vi "Get Package Details.vi"(7 "LabVIEW Web Service Request":refnum<class "Web Request.lvclass">) -> ()   [LabVIEW 2020]
uses:
  <vilib>/wsapi/Web Request.lvclass
  Libraries/Packages/Repo_class/Repo.lvclass/Repo.ctl
  Libraries/Packages/Package_class/Package.lvclass/Package.ctl
  Libraries/Packages/Package Version_class/Package Version.lvclass/Package Version.ctl
  Libraries/Packages/Package Version_class/Read Version.vi
  Libraries/Packages/Package_class/Read Versions.vi
  Libraries/Packages/Package_class/Read Name.vi
  Libraries/Packages/Repo_class/Read Packages.vi
  Libraries/WSsupport/GV_Repos.vi
  Libraries/Packages/Package_class/Package.lvclass
  Libraries/Packages/Package Version_class/Package Version.lvclass
  Libraries/WSsupport/WSsupport.lvlib
  Libraries/ServerErrors/ServerErrors.lvlib
  Libraries/Packages/Repo_class/Repo.lvclass
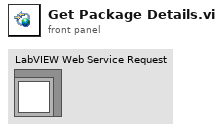
[diagram p1: front panel]
types:
  T1 = typedef "ServerErrors.lvlib/Error Message--cluster.ctl" = cluster{"HTTP Code":i32, "JSON Response":cluster{"error":string, "reason":string}}
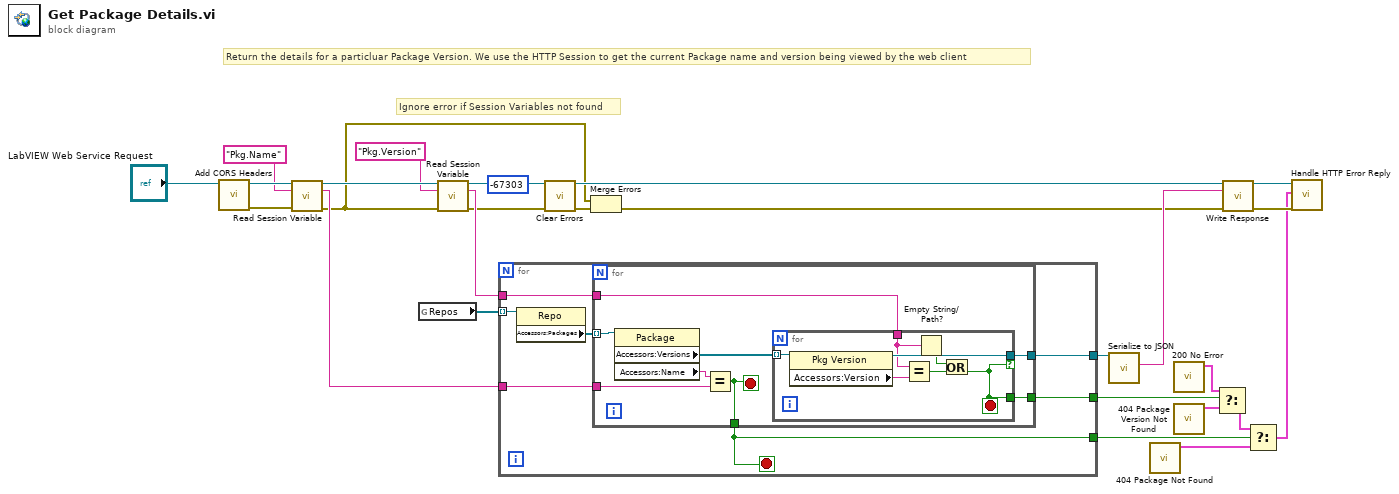
[diagram p0: block diagram]
diagram:
  # "Ignore error if Session Variables not found"
  # "Return the details for a particluar Package Version. We use the HTTP Session to get the current Package name and version being viewed by the web client"
  n1 = call "Add CORS Headers.vi"("LabVIEW Web Service Request"="LabVIEW Web Service Request") -> ("error out"=w24:errorcluster, "LabVIEW Web Service Request out"=w25:refnum<class "Web Request.lvclass">)  [unwired: 9 in]
  n2 = call <vilib>:"Read Session Variable.vi"("LabVIEW Web Service Request"=w25, "key"="Pkg.Name", "error in (no error)"=w24) -> ("LabVIEW Web Service Request out"=w22:refnum<class "Web Request.lvclass">, "value"=w19:string, "error out"=w1:errorcluster)  [unwired: 10 in]
  n3 = global read "GV_Repos.vi" "Repos"() -> (w20:refnum<class "Repo.lvclass">[])
  n4 = call <vilib>:"Read Session Variable.vi"("LabVIEW Web Service Request"=w22, "key"="Pkg.Version", "error in (no error)"=w1) -> ("LabVIEW Web Service Request out"=w16:refnum<class "Web Request.lvclass">, "value"=w18:string, "error out"=w15:errorcluster)  [unwired: 10 in]
  n5 = for {
    tunnel: w20 -> [w33] mode=indexing
    tunnel: w19 -> [w31]
    tunnel: w18 -> [w30]
    tunnel: [w29] -> w17
    tunnel: [w27] -> w11
    tunnel: [w28] -> w9
    stop <- w27 stop-if-true
    n6 = property class="Repo"(reference=w33) -> ("Accessors:Packages"=w32:refnum<class "Package.lvclass">[])  [unwired: 1 in, 2 out]
    n7 = for {
      tunnel: w32 -> [w41] mode=indexing
      tunnel: w31 -> [w39]
      tunnel: [w35] -> w27
      tunnel: w30 -> [w37]
      tunnel: [w36] -> w29
      tunnel: [w34] -> w28
      stop <- w35 stop-if-true
      n8 = property class="Package"(reference=w41) -> ("Accessors:Versions"=w38:refnum<class "Package Version.lvclass">[], "Accessors:Name"=w40:string)  [unwired: 1 in, 2 out]
      n9 = Equal?(x=w40, y=w39) -> (x = y?=w35:bool)
      n10 = for {
        tunnel: w38 -> [w48] mode=indexing
        tunnel: w37 -> [w43]
        tunnel: [w46] -> w36 if=w44
        tunnel: [w44] -> w34
        stop <- w44 stop-if-true
        n11 = property class="Pkg Version"(reference=w48) -> (reference out=w46:refnum<class "Package Version.lvclass">, "Accessors:Version"=w47:string)  [unwired: 1 in, 1 out]
        n12 = Equal?(x=w43, y=w47) -> (x = y?=w45:bool)
        n13 = Empty String/Path?(string/path=w43) -> (empty?=w42:bool)
        n14 = Or(x=w42, y=w45) -> (x .or. y?=w44:bool)
      }
    }
  }
  n15 = call <vilib>:"Clear Errors.vi"("error in (no error)"=w15, "specific error code to clear (0: all)"=-67303) -> ("error out"=w4:errorcluster)  [unwired: 4 in, 1 out]
  n16 = Merge Errors(w1, w4) -> (w2:errorcluster)
  n17 = call-dynamic "Serialize to JSON.vi"("Pkg Details in"=w17) -> ("JSON string"=w14:string)  [unwired: 7 in, 3 out]
  n18 = call "404 Package Not Found.vi"() -> ("error"=w10:T1)  [unwired: 11 in]
  n19 = call "200 No Error.vi"() -> ("no error"=w8:T1)  [unwired: 11 in]
  n20 = call "404 Package Version Not Found.vi"() -> ("error"=w7:T1)  [unwired: 11 in]
  n21 = Select(t=w8, s=w9, f=w7) -> (s? t:f=w6:T1)
  n22 = call <vilib>:"Write Response.vi"("LabVIEW Web Service Request"=w16, "response string"=w14, "error in (no error)"=w2) -> ("LabVIEW Web Service Request out"=w13:refnum<class "Web Request.lvclass">, "error out"=w12:errorcluster)  [unwired: 11 in]
  n23 = Select(t=w6, s=w11, f=w10) -> (s? t:f=w5:T1)
  n24 = call "Handle HTTP Error Reply.vi"("error in (no error)"=w12, "HTTP Status Code"=w5, "Web Request in"=w13) -> ()  [unwired: 8 in, 1 out]
